vi "Script Msg Init VI.vi"(8 "error in":errorcluster, 9 "Ref.Init VI":refnum<vi>, 10 "Conpane Map":T1(c390)) -> (0 "error out":errorcluster)   [LabVIEW 2025, in "_Msg Rescript.lvlib" / "_Msg Rescript.lvclass"]
uses:
  _Msg Rescript.lvclass
  _Msg Rescript.lvclass/_Msg Rescript.ctl
  <vilib>/Utility/traverseref.llb/TRef TravTarget.ctl
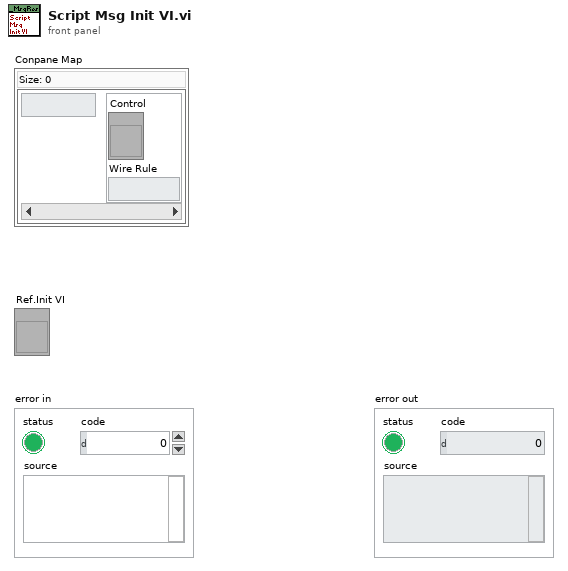
[diagram p1: front panel]
types:
  T1 = map{i32, cluster{"Control":refnum<vi>, "Wire Rule":enum16{"Invalid Wire Rule", "Required", "Recommended", "Optional", "Dynamic Dispatch"}}}
  T2 = typedef "TRef TravTarget.ctl" = enum16{"FP", "BD", "Other"}
  T3 = enum16{"Invalid Wire Rule", "Required", "Recommended", "Optional", "Dynamic Dispatch"}
  T4 = cluster{"Control":refnum<vi>, "Wire Rule":enum16{"Invalid Wire Rule", "Required", "Recommended", "Optional", "Dynamic Dispatch"}}
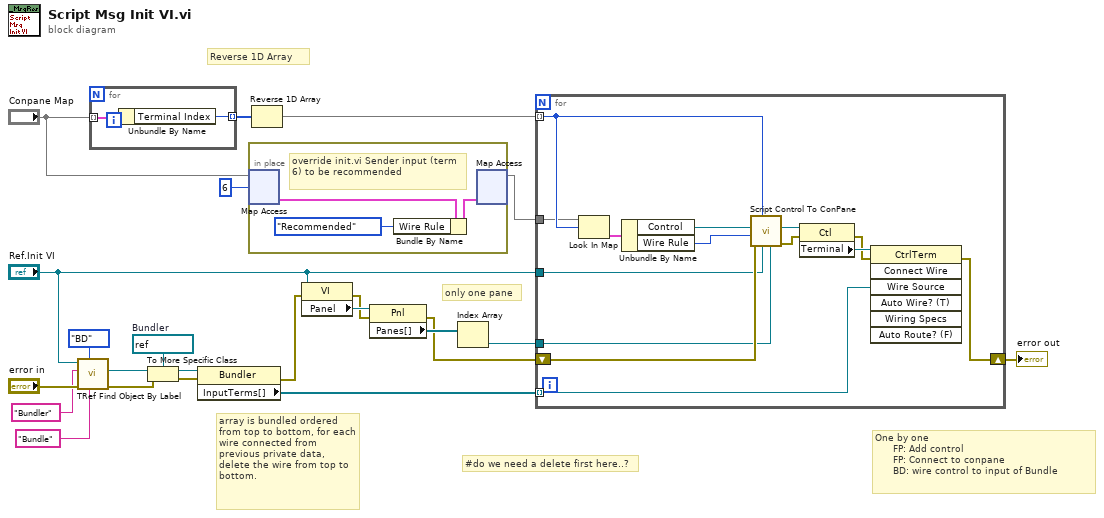
[diagram p0: block diagram]
diagram:
  w10 = refnum<vi> refnum  # Bundler
  # "#do we need a delete first here..?"
  # "array is bundled ordered from top to bottom, for each wire connected from previous private data, delete the wire from top to bottom."
  # "Reverse 1D Array"
  # "One by one\n      FP: Add control\n      FP: Connect to conpane\n      BD: wire control to input of Bundle"
  # "only one pane"
  n1 = call <vilib>:"TRef Find Object By Label.vi"("Label"="Bundle", "Traverse Target"=TRef_TravTarget."BD", "error in (no error)"="error in", "Class Name"="Bundler", "VI Ref"="Ref.Init VI") -> ("error out"=w14:errorcluster, "Found Obj Ref"=w13:refnum<vi>)  [unwired: 3 in, 2 out]
  n2 = for {
    tunnel: "Conpane Map" -> [w25] mode=indexing
    tunnel: [w24] -> w23 mode=indexing
    n3 = Unbundle By Name(w25) -> ("Terminal Index"=w24:i32)
  }
  n4 = To More Specific Class(target class=w10, reference=w13, error in=w14) -> (specific class reference=w8:refnum<vi>, error out=w7:errorcluster)
  n5 = property class="Bundler"(reference=w8, error in=w7) -> (error out=w19:errorcluster, "InputTerms[]"=w3:refnum<vi>[])  [unwired: 1 out]
  n6 = in-place {
    # "override init.vi Sender input (term 6) to be recommended"
    n7 = in-place-map #1("Conpane Map", 6 ("Terminal Index")) -> (w28:T4)  [unwired: 1 in, 1 out]
    n8 = Bundle By Name(cluster=w28, "Wire Rule"=T3."Recommended") -> (w27:T4)
    n9 = in-place-map #1(w27) -> (w2:T1)  [unwired: 1 in, 2 out]
  }
  n10 = Reverse 1D Array(array=w23) -> (reversed array=w22:i32[])
  n11 = property class="VI"(reference="Ref.Init VI", error in=w19) -> (error out=w18:errorcluster, "Panel"=w21:refnum<vi>)  [unwired: 1 out]
  n12 = property class="Pnl"(reference=w21, error in=w18) -> (error out=w17:errorcluster, "Panes[]"=w20:refnum<vi>[])  [unwired: 1 out]
  n13 = Index Array(array=w20) -> (element=w16:refnum<vi>)  [unwired: 1 in]
  n14 = for {
    tunnel: w22 -> [w30] mode=indexing
    tunnel: w2 -> [w29]
    tunnel: w16 -> [w35]
    tunnel: "Ref.Init VI" -> [w34]
    tunnel: w3 -> [w41] mode=indexing
    shift-right: [w39] -> w5
    shift-left: w17 -> [w36]
    n15 = Look In Map(map=w29, key=w30) -> (value=w33:T4)  [unwired: 1 in, 1 out]
    n16 = Unbundle By Name(w33) -> ("Control"=w32:refnum<vi>, "Wire Rule"=w31:T3)
    n17 = call "Script Control To ConPane.vi"("Pane"=w35, "VI Ref"=w34, "Terminal Index"=w30, "error in"=w36, "Wire Rule"=w31, "Control"=w32) -> ("error out"=w37:errorcluster, "Control"=w38:refnum<vi>)  [unwired: 4 in]
    n18 = property class="Ctl"(reference=w38, error in=w37) -> (error out=w40:errorcluster, "Terminal"=w42:refnum<vi>)  [unwired: 1 out]
    n19 = invoke class="CtrlTerm" method="Connect Wire"(reference=w42, error in=w40, "Wire Source"=w41) -> (error out=w39:errorcluster)  [unwired: 4 in, 6 out]
  }
  "error out" <- w5
